vi "Check Trigger Conditions.vi"(6 "Force Trigger?":bool, 8 "error in (no error)":errorcluster, 10 "Waveform Data In":waveform(dbl)[](array[waveform]), 11 "Logging Configuration In":T1) -> (0 "error out":errorcluster, 1 "Trigger Conditions Met?":bool, 2 "Waveform Data Out (copy)":waveform(dbl)[](array[waveform]), 3 "Logging Configuration Out":T1)   [LabVIEW 2024, in "Logging.lvlib"]
doc: "Given the Logging Configuration, Waveform Data, and Force Trigger information, return true if a trigger has been detected."
uses:
  Logging.lvlib
  Logging Configuration.ctl
  <vilib>/Analysis/NI_AALPro.lvlib
panel:
  # "(Scroll up to see Logging Configuration Controls)"
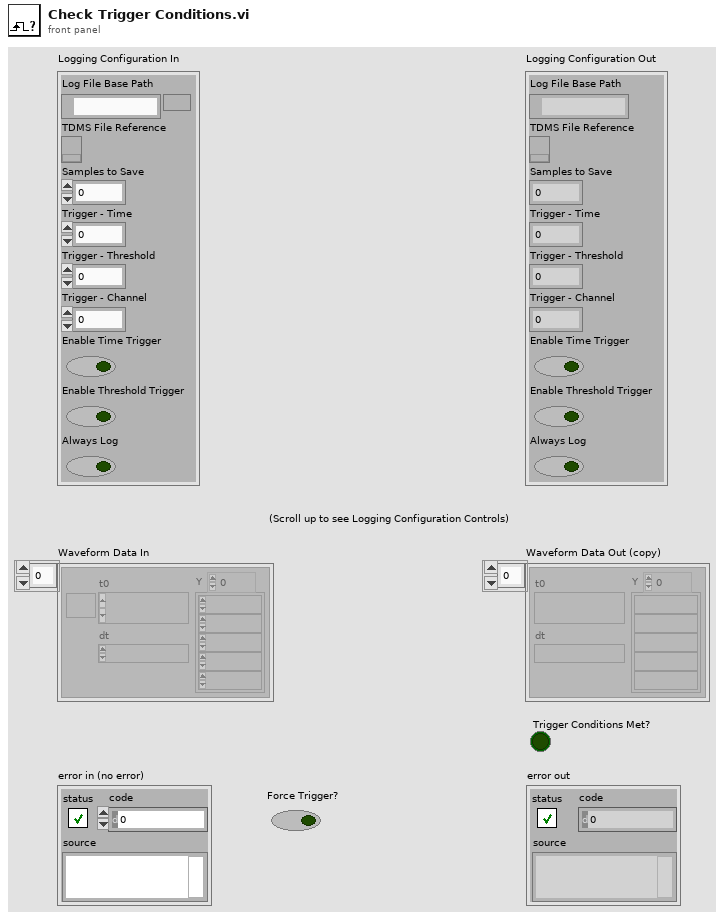
[diagram p1: front panel]
types:
  T1 = typedef "Logging.lvlib/Logging Configuration.ctl" = cluster{"Log File Base Path":path, "TDMS File Reference":refnum<k34>, "Samples to Save":u32, "Trigger - Time":u32, "Trigger - Threshold":dbl, "Trigger - Channel":u32, "Enable Time Trigger":bool, "Enable Threshold Trigger":bool, "Always Log":bool}
  T2 = typedef "LVDateTimeRec.ctl" = cluster{"fractional second":dbl, "second":i32, "minute":i32, "hour":i32, "day of month":i32, "month":i32, "year":i32, "day of week":i32, "day of year":i32, "DST":i32}
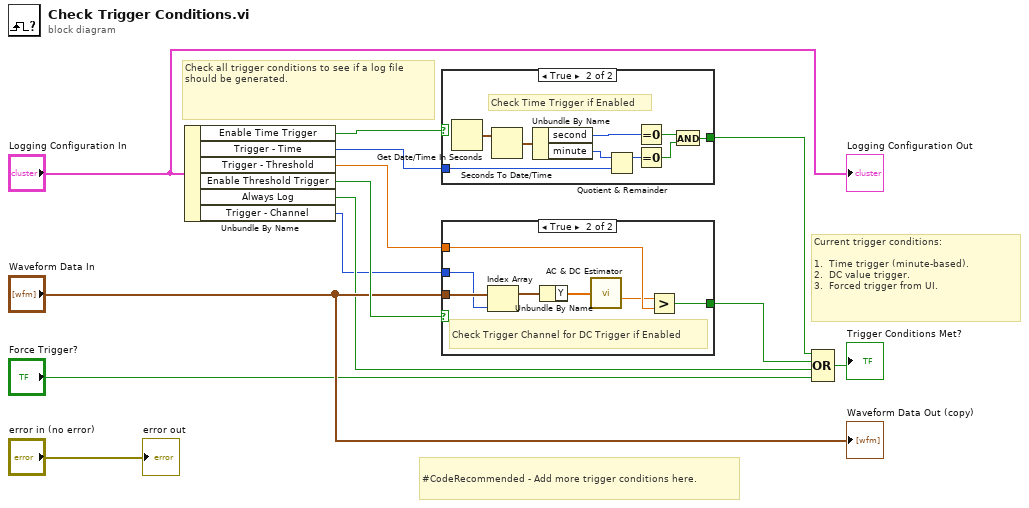
[diagram p0: block diagram]
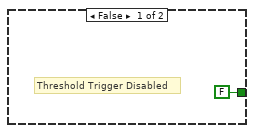
[diagram p2: hidden frame]
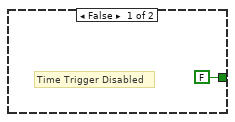
[diagram p3: hidden frame]
diagram:
  # "Check all trigger conditions to see if a log file should be generated."
  # "Current trigger conditions:\n\n1.  Time trigger (minute-based).\n2.  DC value trigger.\n3.  Forced trigger from UI."
  # "#CodeRecommended - Add more trigger conditions here."
  n1 = Unbundle By Name("Logging Configuration In") -> ("Enable Time Trigger"=w8:bool, "Trigger - Time"=w9:u32, "Trigger - Threshold"=w10:dbl, "Enable Threshold Trigger"=w7:bool, "Always Log"=w4:bool, "Trigger - Channel"=w1:u32)
  n2 = case shown="True" w8 {
    tunnel: [FALSE w16] -> w11
    tunnel: w9 -> [_ w15]
    frame False {
      # "Time Trigger Disabled"
    }
    frame True {
      # "Check Time Trigger if Enabled"
      n3 = Get Date/Time In Seconds() -> (seconds since 1Jan1904=w20:timestamp)
      n4 = Seconds To Date/Time(time stamp (now)=w20) -> (date time rec=w23:T2)  [unwired: 1 out]
      n5 = Unbundle By Name(w23) -> ("second"=w22:i32, "minute"=w19:i32)
      n6 = Quotient & Remainder(x=w19, y=w15) -> (x-y*floor(x/y)=w18:u32)  [unwired: 1 out]
      n7 = Equal To 0?(x=w22) -> (x = 0?=w21:bool)
      n8 = Equal To 0?(x=w18) -> (x = 0?=w17:bool)
      n9 = And(x=w21, y=w17) -> (x .and. y?=w16:bool)
    }
  }
  n10 = case shown="True" w7 {
    tunnel: "Waveform Data In" -> [_ w27]
    tunnel: [FALSE w28] -> w13
    tunnel: w10 -> [_ w31]
    tunnel: w1 -> [_ w25]
    frame False {
      # "Threshold Trigger Disabled"
    }
    frame True {
      # "Check Trigger Channel for DC Trigger if Enabled"
      n11 = Index Array(array=w27, index=w25) -> (element=w26:waveform(dbl))
      n12 = Unbundle By Name(w26) -> ("Y"=w30:dbl[])
      n13 = call <vilib>:"AC & DC Estimator.vi"("Signal (V)"=w30) -> ("DC estimate (V)"=w29:dbl)  [unwired: 1 out]
      n14 = Greater?(x=w29, y=w31) -> (0:w28:bool)
    }
  }
  n15 = Compound Arithmetic op=OR(w11, w13, w4, "Force Trigger?") -> (→"Trigger Conditions Met?":bool)
  "error out" <- "error in (no error)"
  "Waveform Data Out (copy)" <- "Waveform Data In"
  "Logging Configuration Out" <- "Logging Configuration In"
